vi "get type info.vi"(11 "Type in":T1) -> (0 "Offset":u16, 1 "Group GUID":string, 2 "Type GUID":string)   [LabVIEW 2021, in "Modbus Master System Explorer.lvlib"]
uses:
  Modbus Master System Explorer.lvlib
  Modbus Type.ctl
  Shared/Constants.vi
  Shared/Modbus Master Shared.lvlib
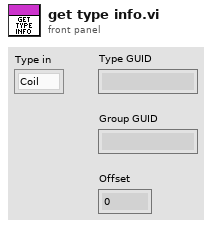
[diagram p1: front panel]
types:
  T1 = typedef "Modbus Master Shared.lvlib/Modbus Type.ctl" = enum16{"Coil", "Discrete Input", "Holding Register", "Input Register"}
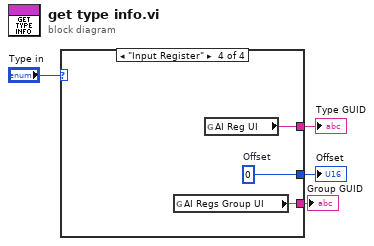
[diagram p0: block diagram]
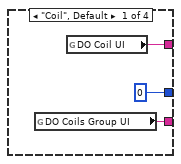
[diagram p2: hidden frame]
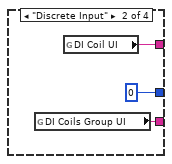
[diagram p3: hidden frame]
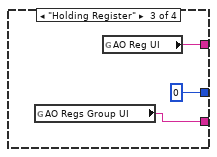
[diagram p4: hidden frame]
diagram:
  n1 = case shown="\"Input Register\"" "Type in" {
    tunnel: [w7 w10 w13 w16] -> w2
    tunnel: [u16 0 ("Offset") u16 0 ("Offset") u16 0 ("Offset") w15] -> w4
    tunnel: [w5 w8 w11 w14] -> w1
    frame "Coil", Default {
      n2 = global read "Constants.vi" "DO Coils Group UI"() -> (w5:string)
      n3 = global read "Constants.vi" "DO Coil UI"() -> (w7:string)
    }
    frame "Discrete Input" {
      n4 = global read "Constants.vi" "DI Coils Group UI"() -> (w8:string)
      n5 = global read "Constants.vi" "DI Coil UI"() -> (w10:string)
    }
    frame "Holding Register" {
      n6 = global read "Constants.vi" "AO Regs Group UI"() -> (w11:string)
      n7 = global read "Constants.vi" "AO Reg UI"() -> (w13:string)
    }
    frame "Input Register" {
      w15 = u16 0  # Offset
      n8 = global read "Constants.vi" "AI Regs Group UI"() -> (w14:string)
      n9 = global read "Constants.vi" "AI Reg UI"() -> (w16:string)
    }
  }
  "Offset" <- w4
  "Type GUID" <- w2
  "Group GUID" <- w1
